vi "JSON Generator.vi"(8 "error in (no error)":errorcluster, 10 "ECU":refnum<k21>="GIP\ncan_messages_818", 11 "XNET Database":refnum<k21>="GIP_CAN_Database") -> (0 "error out":errorcluster, 1 "Rx Sigs":refnum<k21>[](array[refnum]), 2 "Tx Sigs":refnum<k21>[](array[refnum]), 3 "JSON":string="{\n  \"CAN_Rx\":{\n    \"GIP_GetPartNumber.lChar0\":0,\n    \"GIP_GetPartNumber.lChar1\":1,\n    \"GIP_GetPartNumber.lChar2\":2,\n    \"GIP_GetPartNumber.lChar3\":3,\n    \"GIP_GetPartNumber.lChar4\":4,\n    \"GIP_GetPartNumber.lChar5\":5,\n    \"GIP_GetPartNumber.lChar6\":6,\n    \"GIP_GetPartNumber.lChar7\":7,\n    \"GIP_GetPartNumber.rChar0\":8,\n    \"GIP_GetPartNumber.rChar1\":9,\n    \"GIP_GetSerialNumber.vendorChar0\":10,\n    \"GIP_GetSerialNumber.vendorChar1\":11,\n    \"GIP_GetSerialNumber.vendorChar2\":12,\n    \"GIP_GetSerialNumber.weekAndSerial\":13,\n    \"GIP_Grid_ActiveEnergyExported.GIP_Grid_ActiveEnergyExported_L1\":14,\n    \"GIP_Grid_ActiveEnergyExported.GIP_Grid_ActiveEnergyExported_L2\":15,\n    \"GIP_Grid_ActiveEnergyImported.GIP_Grid_ActiveEnergyImported_L1\":16,\n    \"GIP_Grid_ActiveEnergyImported.GIP_Grid_ActiveEnergyImported_L2\":17,\n    \"GIP_Grid_Power.GIP_Grid_ActivePower_L1\":18,\n    \"GIP_Grid_Power.GIP_Grid_ActivePower_L2\":19,\n    \"GIP_Grid_Power.GIP_Grid_ReactivePower_L1\":20,\n    \"GIP_Grid_Power.GIP_Grid_ReactivePower_L2\":21,\n    \"GIP_Grid_TotalActiveEnergy.GIP_Grid_TotalActiveEnergyExported\":22,\n    \"GIP_Grid_TotalActiveEnergy.GIP_Grid_TotalActiveEnergyImported\":23,\n    \"GIP_Load_ActiveEnergyExported.GIP_Load_ActiveEnergyExported_L1\":24,\n    \"GIP_Load_ActiveEnergyExported.GIP_Load_ActiveEnergyExported_L2\":25,\n    \"GIP_Load_ActiveEnergyImported.GIP_Load_ActiveEnergyImported_L1\":26,\n    \"GIP_Load_ActiveEnergyImported.GIP_Load_ActiveEnergyImported_L2\":27,\n    \"GIP_Load_Power.GIP_Load_ActivePower_L1\":28,\n    \"GIP_Load_Power.GIP_Load_ActivePower_L2\":29,\n    \"GIP_Load_Power.GIP_Load_ReactivePower_L1\":30,\n    \"GIP_Load_Power.GIP_Load_ReactivePower_L2\":31,\n    \"GIP_Load_TotalActiveEnergy.GIP_Load_TotalActiveEnergyExported\":32,\n    \"GIP_Load_TotalActiveEnergy.GIP_Load_TotalActiveEnergyImported\":33,\n    \"GIP_Status.GIP_Relay_State\":34,\n    \"GIP_Status.GIP_State\":35\n  },\n  \"CAN_Tx\":{\n    \"GIP_ManufacturingControl.ESP32Comms\":0,\n    \"GIP_ManufacturingControl.FaultLED\":1,\n    \"GIP_ManufacturingControl.Relay\":2,\n    \"GIP_ManufacturingControl.ST8500Comms\":3,\n    \"GIP_ManufacturingControl.StatusLED\":4,\n    \"GIP_SetPartNumber.lChar0\":5,\n    \"GIP_SetPartNumber.lChar1\":6,\n    \"GIP_SetPartNumber.lChar2\":7,\n    \"GIP_SetPartNumber.lChar3\":8,\n    \"GIP_SetPartNumber.lChar4\":9,\n    \"GIP_SetPartNumber.lChar5\":10,\n    \"GIP_SetPartNumber.lChar6\":11,\n    \"GIP_SetPartNumber.lChar7\":12,\n    \"GIP_SetPartNumber.rChar0\":13,\n    \"GIP_SetPartNumber.rChar1\":14,\n    \"GIP_SetSerialNumber.vendorChar0\":15,\n    \"GIP_SetSerialNumber.vendorChar1\":16,\n    \"GIP_SetSerialNumber.vendorChar2\":17,\n    \"GIP_SetSerialNumber.weekAndSerial\":18,\n    \"GIP_SetTestedFlag.GIP_TestedFlag\":19,\n    \"GIP_TestMode.GIP_TestModeFlag\":20\n  }\n}")   [LabVIEW 2021, in "CAN GIP.lvlib"]
uses:
  CAN GIP.lvlib
  <vilib>/JDP Science/JSONtext/Get all Object Items.vi
  <vilib>/JDP Science/JSONtext/Set Multiple Object Items.vi
  <resource>/objmgr/xnet.rc
  <vilib>/JDP Science/JSONtext/JSONtext.lvlib
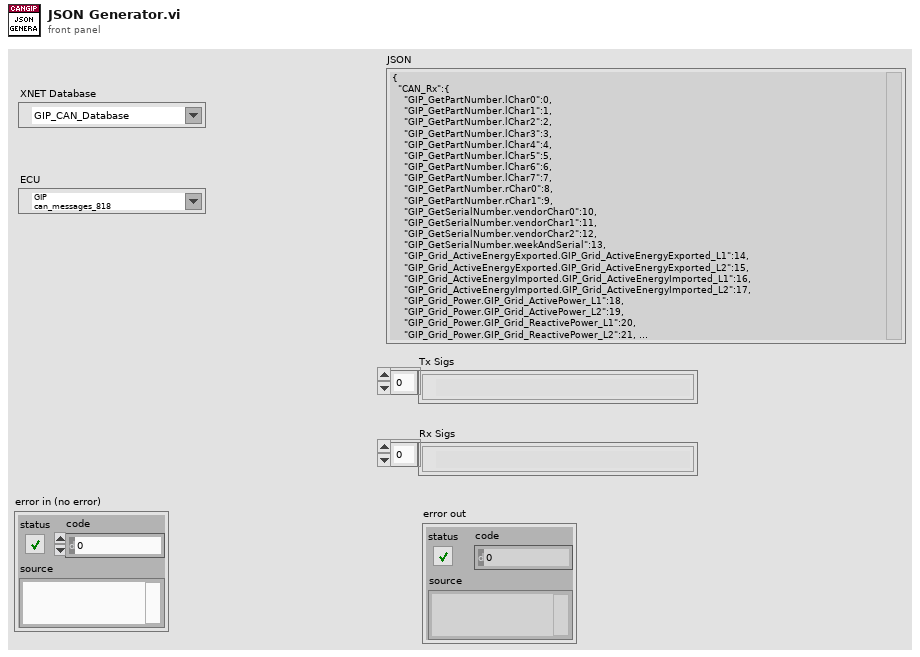
[diagram p1: front panel]
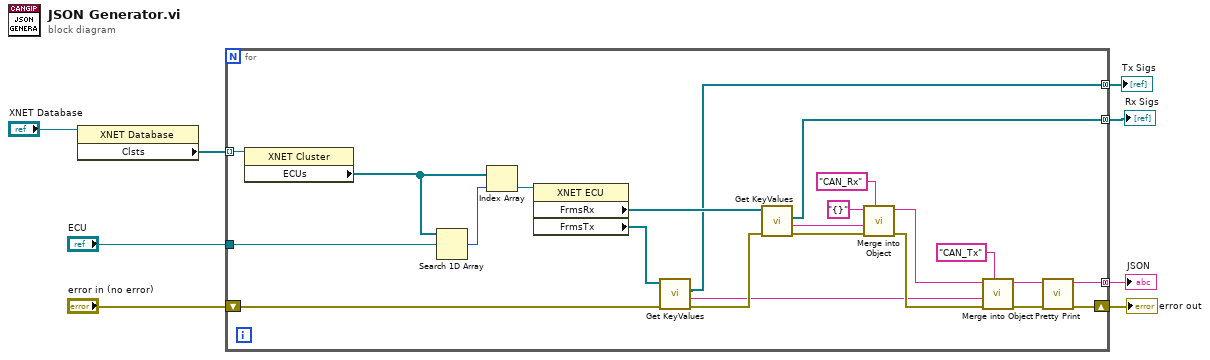
[diagram p0: block diagram]
diagram:
  n1 = property class="XNET Database"(reference="XNET Database") -> ("Clsts"=w7:refnum<k21>[])  [unwired: 1 in, 2 out]
  n2 = for {
    tunnel: w7 -> [w11] mode=indexing
    shift-right: [w25] -> w5
    shift-left: "error in (no error)" -> [w29]
    tunnel: [w27] -> w4 mode=concatenating
    tunnel: [w22] -> w3 mode=concatenating
    tunnel: [w21] -> w2 mode=concatenating
    tunnel: "ECU" -> [w9]
    n3 = property class="XNET Cluster"(reference=w11) -> ("ECUs"=w10:refnum<k21>[])  [unwired: 1 in, 2 out]
    n4 = Search 1D Array(1D array=w10, element=w9) -> (index of element=w31:i32)  [unwired: 1 in]
    n5 = Index Array(array=w10, index=w31) -> (element=w30:refnum<k21>)
    n6 = property class="XNET ECU"(reference=w30) -> ("FrmsRx"=w24:refnum<k21>[], "FrmsTx"=w23:refnum<k21>[])  [unwired: 1 in, 2 out]
    n7 = call "Get KeyValues.vi"("error in (no error)"=w29, "Frames"=w23) -> ("error out"=w20:errorcluster, "<JSON>"=w13:string, "Sigs"=w22:refnum<k21>[])  [unwired: 7 in]
    n8 = call "Get KeyValues.vi"("error in (no error)"=w20, "Frames"=w24) -> ("error out"=w19:errorcluster, "<JSON>"=w12:string, "Sigs"=w21:refnum<k21>[])  [unwired: 7 in]
    n9 = call <vilib>:"Merge into Object.vi"("$Path or Item Name"="CAN_Rx", "error in (no error)"=w19, "JSON Object to Merge"=w12, "JSON"="{}") -> ("error out"=w17:errorcluster, "<JSON>"=w16:string)  [unwired: 5 in]
    n10 = call <vilib>:"Merge into Object.vi"("$Path or Item Name"="CAN_Tx", "error in (no error)"=w17, "JSON Object to Merge"=w13, "JSON"=w16) -> ("error out"=w28:errorcluster, "<JSON>"=w26:string)  [unwired: 5 in]
    n11 = call <vilib>:"Pretty Print.vi"("error in (no error)"=w28, "JSON"=w26) -> ("error out"=w25:errorcluster, "<JSON>"=w27:string)  [unwired: 7 in, 1 out]
  }
  "JSON" <- w4
  "error out" <- w5
  "Tx Sigs" <- w3
  "Rx Sigs" <- w2
